vi "test.vi"(10 "value":variant, 11 "key":string) -> (3 "Variant out":variant)   [LabVIEW 2019]
uses:
  <userlib>/LevyLab/LV-Data/LV-Data/Typedefs/Dictionary--cluster.ctl
  <userlib>/LevyLab/LV-Data/LV-Data/LV-Data.lvclass
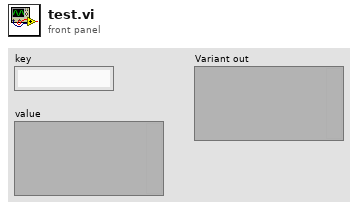
[diagram p1: front panel]
types:
  T1 = typedef "LV-Data.lvclass/Dictionary--cluster.ctl" = cluster{"key":string, "value":variant}
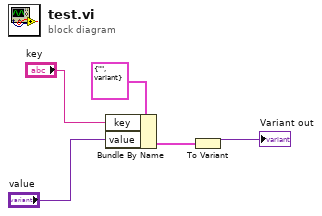
[diagram p0: block diagram]
diagram:
  n1 = Bundle By Name(cluster=T1 {"key"="", "value"=variant} ("param"), "key"="key", "value"="value") -> (w5:T1)
  n2 = To Variant(anything=w5) -> (Variant=→"Variant out":variant)
